vi "Initialize.vi"(8 "error in (no error)":errorcluster, 9 "ID Query":bool, 10 "Reset":bool, 11 "Fluke Hydra 2625A in":refnum<class "Fluke Hydra 2625A.lvclass">) -> (0 "error out":errorcluster, 2 "VISA resource name":refnum<visa-resource-name>, 3 "Fluke Hydra 2625A out":refnum<class "Fluke Hydra 2625A.lvclass">)   [LabVIEW 2016, in "Generic Data Acquisition.lvlib" / "Fluke Hydra.lvlib" / "Fluke Hydra 2625A.lvclass"]
uses:
  Fluke Hydra 2625A.lvclass
  <instrlib>/Fluke 2625A/Fluke 2625A.lvlib
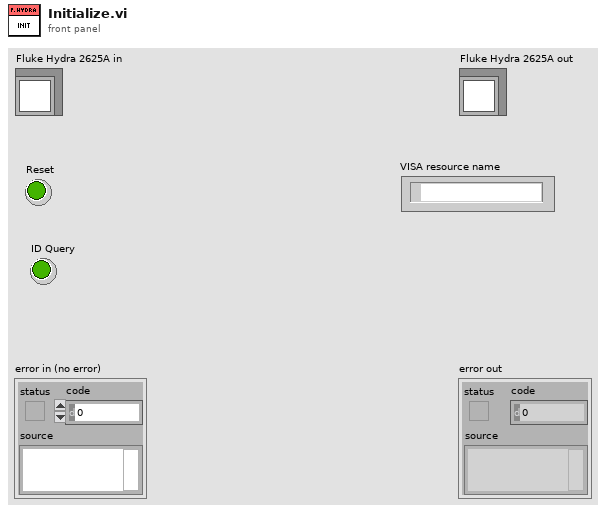
[diagram p1: front panel]
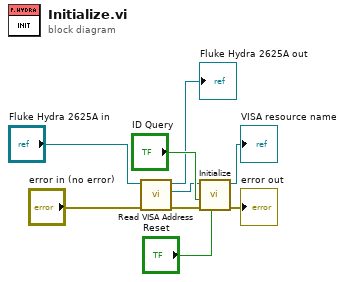
[diagram p0: block diagram]
diagram:
  n1 = call-dynamic "Read VISA Address.vi"("error in (no error)"="error in (no error)", "Generic Device in"="Fluke Hydra 2625A in") -> ("error out"=w3:errorcluster, "VISA Address"=w2:refnum<visa-resource-name>, "Generic Device out"=→"Fluke Hydra 2625A out":refnum<class "Fluke Hydra 2625A.lvclass">)  [unwired: 7 in]
  n2 = call <instrlib>:"Initialize.vi"("Reset"="Reset", "Error"=w3, "Query Instrument"="ID Query", "VISA Resource Name"=w2) -> ("Error Out"=→"error out":errorcluster, "VISA Resource Name Out"=→"VISA resource name":refnum<visa-resource-name>)  [unwired: 5 in, 1 out]
